vi "URI.vi"(11 "IErrorHandler in":refnum<class "AbortHandler JSON.lvclass">) -> (2 "URI":string, 3 "IErrorHandler out":refnum<class "AbortHandler JSON.lvclass">)   [LabVIEW 2020, in "wamplv.lvlib" / "AbortHandler JSON.lvclass"]
uses:
  AbortHandler JSON.lvclass
  AbortHandler JSON.lvclass/AbortHandler JSON.ctl
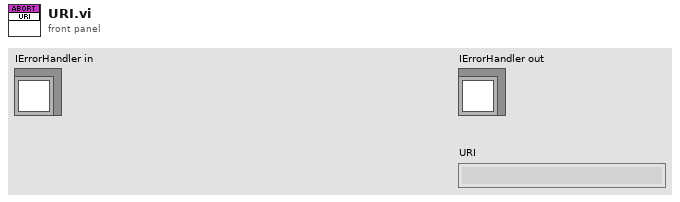
[diagram p1: front panel]
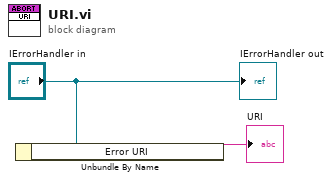
[diagram p0: block diagram]
diagram:
  n1 = Unbundle By Name("IErrorHandler in") -> ("Error URI"=→"URI":string)
  "IErrorHandler out" <- "IErrorHandler in"
